vi "WriteReport.vi"(7 "Diag_Ver":string, 8 "error in (no error)":errorcluster, 9 "StepName":string, 10 "Pass/Fail":bool, 11 "GuiRef":T2={"StringOut"=refnum, "AbortOnFail"=refnum, "SN"=refnum, "SN_Length"=refnum, "TestResult"=refnum, "CycleTime"=refnum, "ErrorCode"=refnum, "UUTStatus"=refnum, "DataBaseEnable?"=refnum, "DUTModel"=refnum, "FixtureID"=refnum, "OperatorID"=refnum, "SNReady"=refnum, "StopSlot"=refnum, "NextStep"=refnum, "PassYeild"=refnum, "Failed"=refnum, "Passed"=refnum, "Tested"=refnum, "TestItemsCtl"={"StepName"="", "TestEnable"=FALSE, "LoopCount"=0, "StopOnFail"=FALSE, "Index"=0, "TestName"="", "通道"="", "参数"="", "TimeStart"=0}, "ProcessBar"=refnum, "Slot"=enum."Slot1", "Row"=3, "States"=refnum, "TestMode"=refnum, "循环次数-DUT"=refnum, "波形图"=refnum, "产品型号"=refnum, "子面板"=refnum, "测试失败项目"=refnum, "测试结果"=refnum, "DUT"=refnum, "Starttime"=refnum, "SlotReady"=refnum, "版本信息"=refnum, "WIFI_1"=refnum, "WIFI_2"=refnum, "直通率"=refnum, "卡1开卡结果"=refnum, "卡2开卡结果"=refnum}) -> (0 "error out":errorcluster caption="error out (no error)", 1 "DBresult":bool, 3 "TestData-NHLD":string[](array[string]))   [LabVIEW 2013]
uses:
  SysControl/Reference.ctl
  SysControl/TestItemsCTL.ctl
  SysControl/Slot.ctl
  SourceCode/PDINFO.ctl
  DataBase/DBPara.ctl
  SourceCode/GlobalValue.vi
  <vilib>/Utility/file.llb/Write To Spreadsheet File (string).vi
panel:
  out "Slot":T1
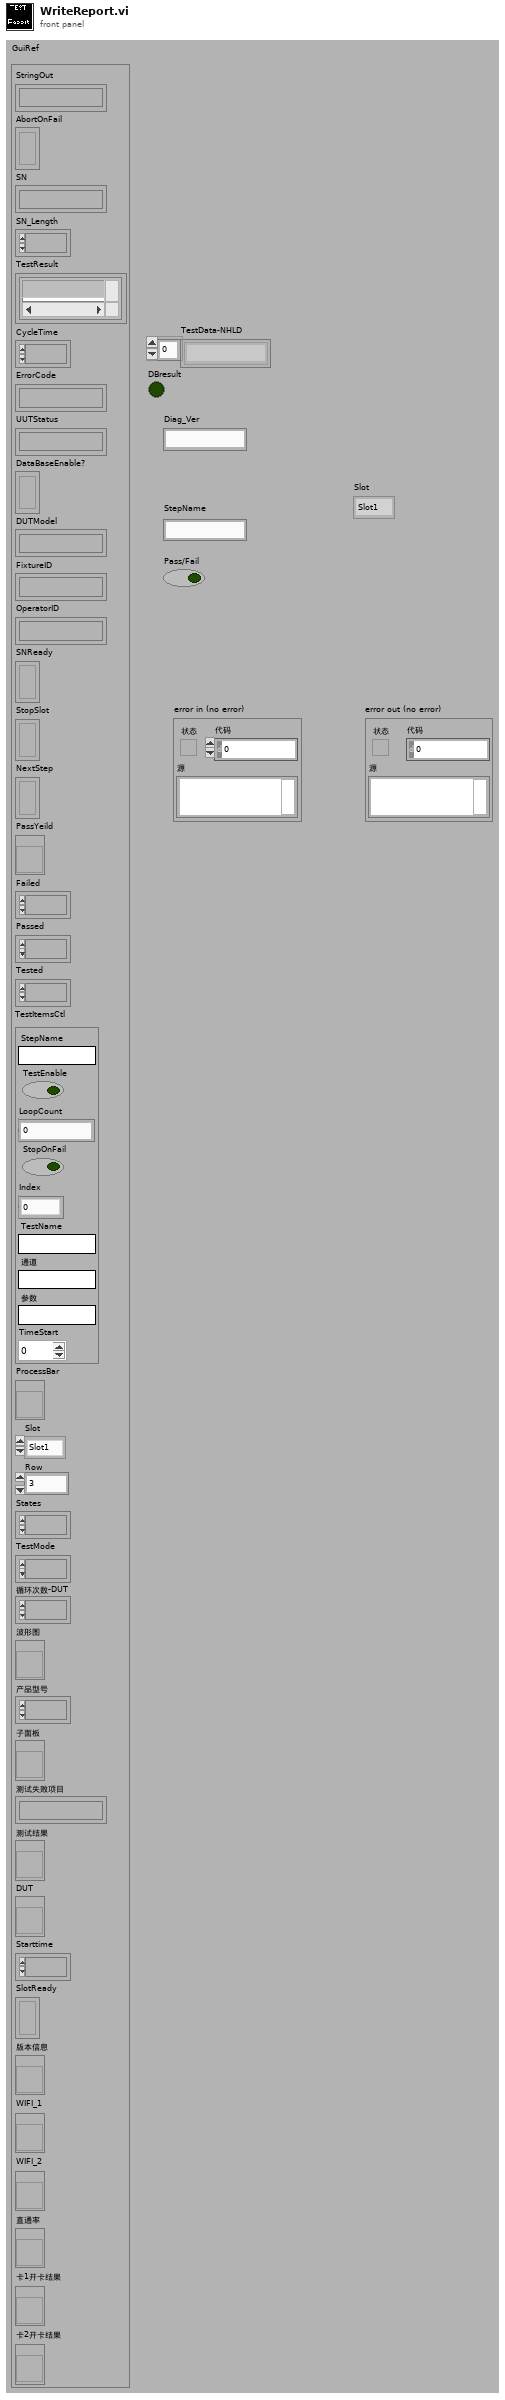
[diagram p1: front panel]
types:
  T1 = typedef "Slot.ctl" = enum16{"Slot1", "Slot2", "Slot3", "Slot4"}
  T2 = typedef "Reference.ctl" = cluster{"StringOut":refnum<vi>, "AbortOnFail":refnum<vi>, "SN":refnum<vi>, "SN_Length":refnum<vi>, "TestResult":refnum<vi>, "CycleTime":refnum<vi>, "ErrorCode":refnum<vi>, "UUTStatus":refnum<vi>, "DataBaseEnable?":refnum<vi>, "DUTModel":refnum<vi>, "FixtureID":refnum<vi>, "OperatorID":refnum<vi>, "SNReady":refnum<vi>, "StopSlot":refnum<vi>, "NextStep":refnum<vi>, "PassYeild":refnum<vi>, "Failed":refnum<vi>, "Passed":refnum<vi>, "Tested":refnum<vi>, "TestItemsCtl":T3, "ProcessBar":refnum<vi>, "Slot":T1, "Row":u32, "States":refnum<vi>, "TestMode":refnum<vi>, "循环次数-DUT":refnum<vi>, "波形图":refnum<vi>, "产品型号":refnum<vi>, "子面板":refnum<vi>, "测试失败项目":refnum<vi>, "测试结果":refnum<vi>, "DUT":refnum<vi>, "Starttime":refnum<vi>, "SlotReady":refnum<vi>, "版本信息":refnum<vi>, "WIFI_1":refnum<vi>, "WIFI_2":refnum<vi>, "直通率":refnum<vi>, "卡1开卡结果":refnum<vi>, "卡2开卡结果":refnum<vi>}
  T3 = typedef "TestItemsCTL.ctl" = cluster{"StepName":string, "TestEnable":bool, "LoopCount":i32, "StopOnFail":bool, "Index":u32, "TestName":string, "通道":string, "参数":string, "TimeStart":u32}
  T4 = enum16{"open", "replace", "create", "open or create", "replace or create", "replace or create with confirmation"}
  T5 = enum16{"Production Mode", "Selection Mode", "Debug Mode", "Loop Mode", "Stop Test"}
  T6 = typedef "PDINFO.ctl" = enum16{"Fw Ver", "HW Ver", "CCID", "WiFiName", "DevID", "SN", "TUID", "CertifID", "PdTime", "Provider", "WiFiPassword", "Imei", "AuthCode", "Reserved1", "Reserved2", "Reserved3"}
  T7 = typedef "DBPara.ctl" = cluster{"DeviceType":string, "PartNumber":string, "TUID":string, "Hw":string, "Sw":string, "PTime":string, "SN":string, "Certid":string, "ICCID":string, "Imei":string, "AuthCode":string, "MAC":string, "Result":string}
  T8 = cluster{"Serial#":string, "TestDate_Time":string, "Operator":string, "TestStation":string, "Fixture#":string, "TestTime":string, "Diag_Ver":string, "Pass_Fail":string}
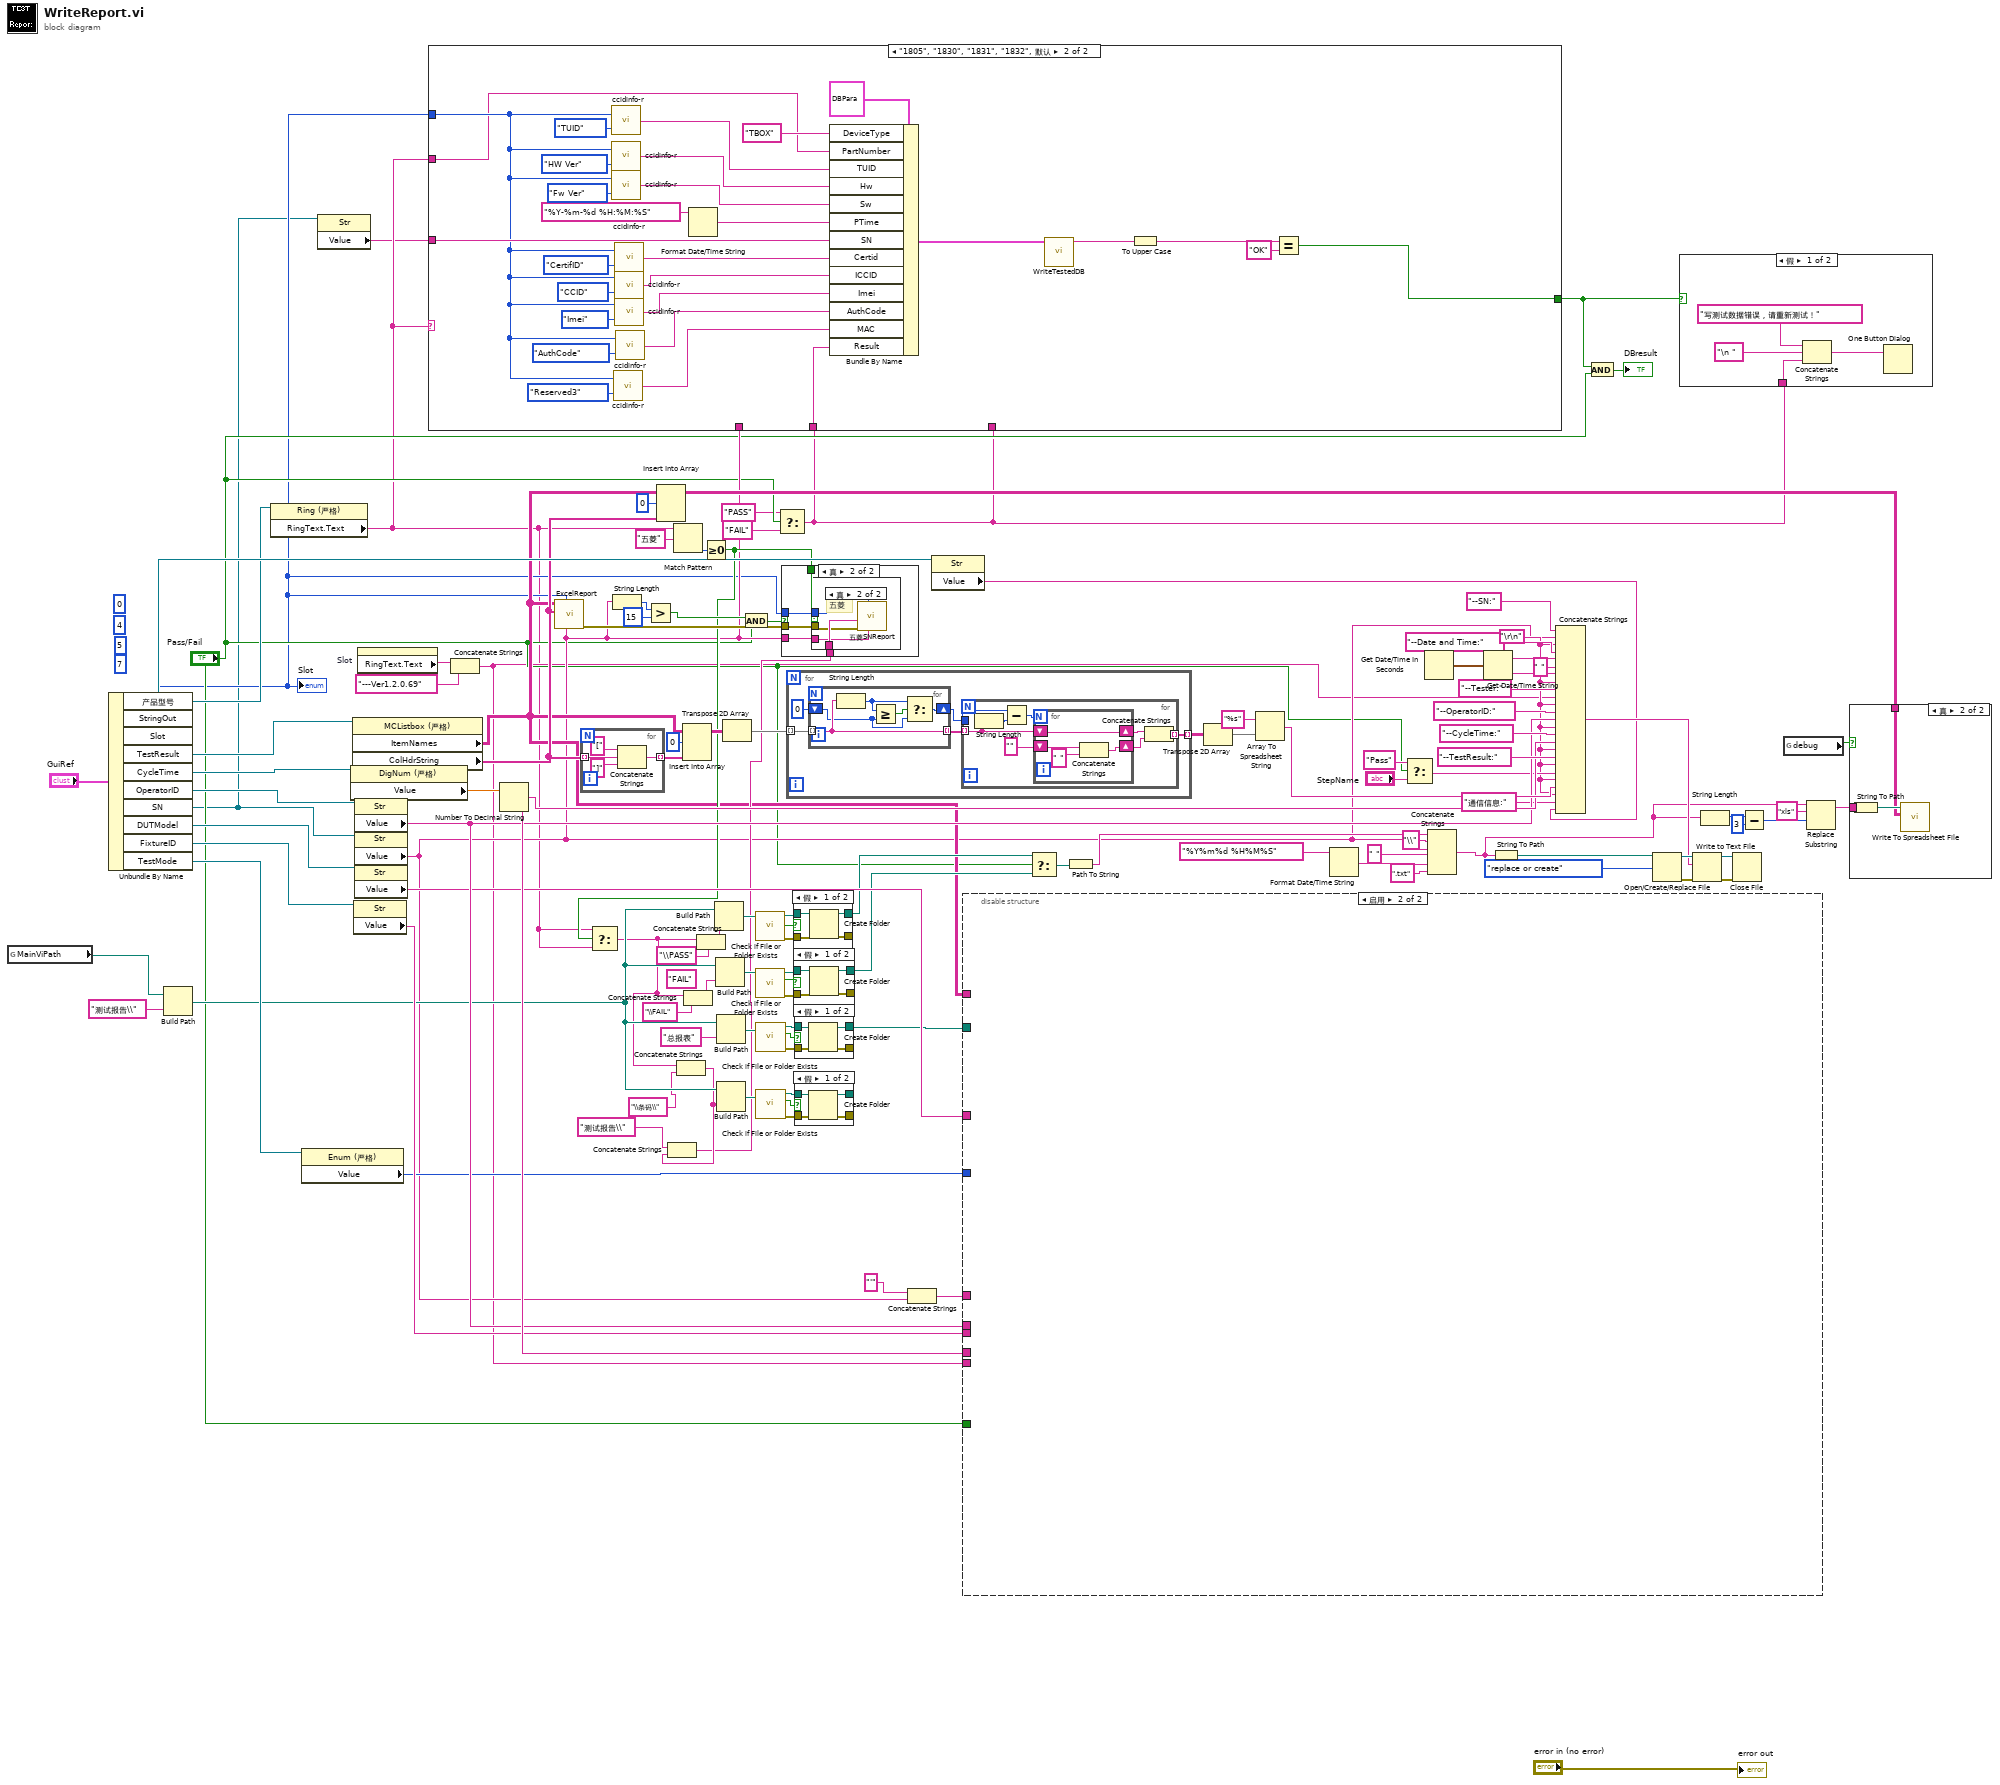
[diagram p0: block diagram]
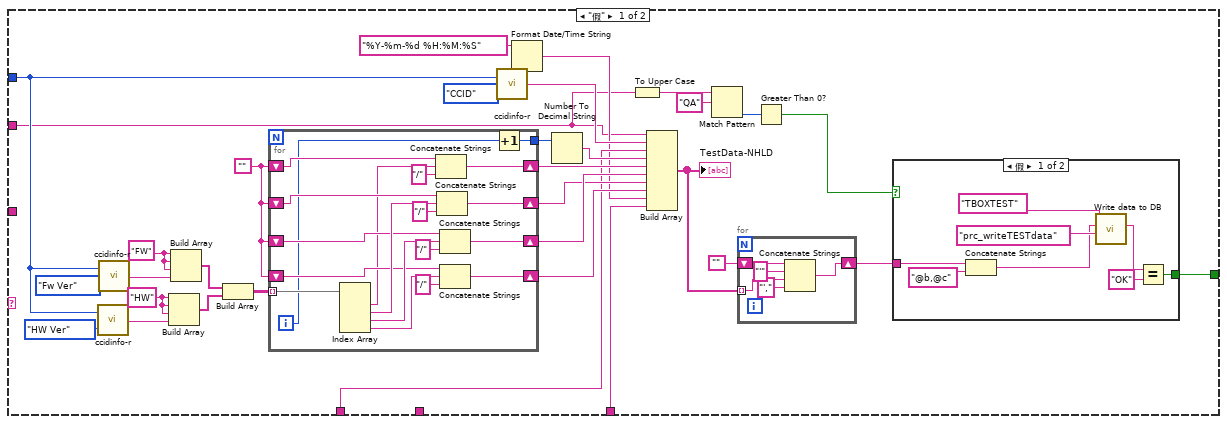
[diagram p2: hidden frame]
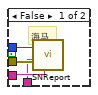
[diagram p7: hidden frame]
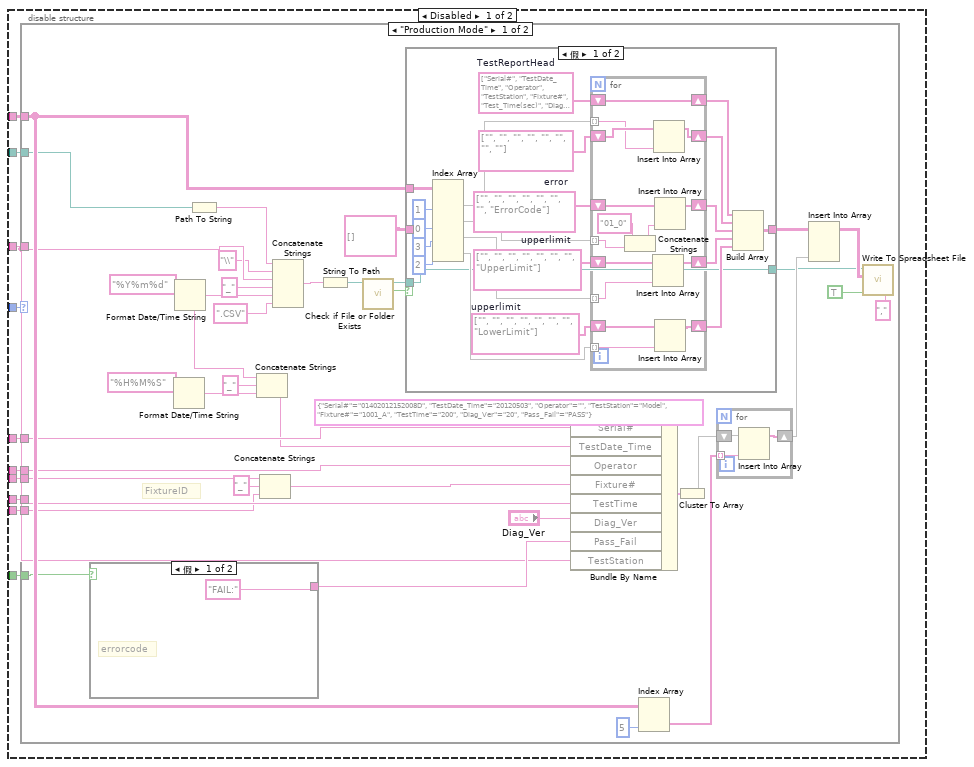
[diagram p9: hidden frame]
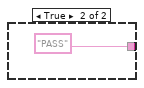
[diagram p10: hidden frame]
diagram:
  (unwired) 7 ("索引")
  (unwired) 5 ("索引")
  (unwired) 4 ("索引")
  (unwired) 0 ("索引")
  (unwired) "FAIL" ("name or relative path")
  w55 = "\r\n"
  n1 = global read "GlobalValue.vi" "MainViPath"() -> (w49:path)
  n2 = Unbundle By Name("GuiRef") -> ("产品型号"=w38:refnum<vi>, "StringOut"=w51:refnum<vi>, "Slot"=w9:T1, "TestResult"=w88:refnum<vi>, "CycleTime"=w87:refnum<vi>, "OperatorID"=w86:refnum<vi>, "SN"=w3:refnum<vi>, "DUTModel"=w85:refnum<vi>, "FixtureID"=w80:refnum<vi>, "TestMode"=w58:refnum<vi>)
  "Slot" <- w9
  n3 = Build Path(base path=w49, name or relative path="测试报告\\" ("名称或相对路径")) -> (appended path=w44:path)
  n4 = property class="Ring (严格)"(reference=w38) -> ("RingText.Text"=w4:string)  [unwired: 1 in, 2 out]
  n5 = property class="Enum (严格)"(reference=w58) -> ("Value"=w57:T5)  [unwired: 1 in, 2 out]
  n6 = property class="Str"(reference=w3) -> ("Value"=w2:string)  [unwired: 1 in, 2 out]
  n7 = property class="DigNum (严格)"(reference=w87) -> ("Value"=w84:dbl)  [unwired: 1 in, 2 out]
  n8 = property class="MCListbox (严格)"(reference=w88) -> ("ItemNames"=w15:string[][], "ColHdrString"=w19:string[])  [unwired: 1 in, 2 out]
  n9 = property class="Str"(reference=w80) -> ("Value"=w79:string)  [unwired: 1 in, 2 out]
  n10 = property class="Str"(reference=w86) -> ("Value"=w83:string)  [unwired: 1 in, 2 out]
  n11 = property class="Str"(reference=w3) -> ("Value"=w14:string)  [unwired: 1 in, 2 out]
  n12 = property class="Str"(reference=w85) -> ("Value"=w82:string)  [unwired: 1 in, 2 out]
  n13 = property on="Slot" class="Enum (严格)"() -> ("RingText.Text"=w7:string)  [unwired: 2 in, 2 out]
  n14 = Concatenate Strings(w7, "---Ver1.2.0.69" ("字符串")) -> (w5:string)
  n15 = Number To Decimal String(number=w84) -> (decimal integer string=w92:string)  [unwired: 1 out]
  n16 = call "ExcelReport.vi"("SN"=w14, "Slot"=w9, "列首字符串"=w19, "TestResults"=w15) -> ("error out"=w43:errorcluster)  [unwired: 7 in]
  n17 = for "For循环" {
    tunnel: w19 -> [w124] mode=indexing
    tunnel: [w122] -> w109 mode=indexing
    n18 = Concatenate Strings("[" ("字符串"), w124, "]" ("字符串")) -> (w122:string)
  }
  n19 = String Length(string=w14) -> (length=w42:i32)
  n20 = Greater?(x=w42, y=15) -> (0:w40:bool)
  n21 = Insert Into Array(array=w15, index (row)=0 ("索引 (行)"), new element=w19) -> (w17:string[][])  [unwired: 1 in]
  n22 = Match Pattern(string=w4, regular expression="五菱" ("正则表达式")) -> (offset past match=w36:i32)  [unwired: 1 in, 3 out]
  n23 = Insert Into Array(array=w15, index (row)=0 ("索引 (行)"), new element=w109) -> (w112:string[][])  [unwired: 1 in]
  n24 = Greater Or Equal To 0?(x=w36) -> (x >= 0?=w35:bool)
  n25 = Select(t=w4, s=w35, f=w4) -> (s? t:f=w29:string)
  n26 = Concatenate Strings(w29, "\\条码\\" ("name or relative path")) -> (w27:string)
  n27 = Concatenate Strings("测试报告\\" ("字符串"), w27) -> (w26:string)
  n28 = Concatenate Strings(w29, "\\FAIL" ("name or relative path")) -> (w31:string)
  n29 = Concatenate Strings(w29, "\\PASS" ("name or relative path")) -> (w34:string)
  n30 = Build Path(base path=w44, name or relative path=w34) -> (appended path=w70:path)
  n31 = Build Path(base path=w44, name or relative path=w31) -> (appended path=w69:path)
  n32 = Build Path(base path=w44, name or relative path="总报表") -> (appended path=w77:path)
  n33 = Build Path(base path=w44, name or relative path=w27) -> (appended path=w46:path)
  n34 = Transpose 2D Array(2D array=w112) -> (transposed array=w120:string[][])
  n35 = And(x=w40, y="Pass/Fail") -> (x .and. y?=w39:bool)
  n36 = call <vilib>:"Check if File or Folder Exists.vi"("path"=w70) -> ("error out"=w74:errorcluster, "file or folder exists?"=w60:bool, "dup path"=w73:path)  [unwired: 1 in, 7 out]
  n37 = call <vilib>:"Check if File or Folder Exists.vi"("path"=w69) -> ("error out"=w71:errorcluster, "file or folder exists?"=w59:bool, "dup path"=w72:path)  [unwired: 1 in, 7 out]
  n38 = call <vilib>:"Check if File or Folder Exists.vi"("path"=w77) -> ("error out"=w76:errorcluster, "file or folder exists?"=w61:bool, "dup path"=w78:path)  [unwired: 1 in, 7 out]
  n39 = call <vilib>:"Check if File or Folder Exists.vi"("path"=w46) -> ("error out"=w47:errorcluster, "file or folder exists?"=w48:bool, "dup path"=w45:path)  [unwired: 1 in, 7 out]
  n40 = Select(t="PASS" ("元素"), s="Pass/Fail", f="FAIL" ("元素")) -> (s? t:f=w1:string)
  n41 = case shown="\"1805\", \"1830\", \"1831\", \"1832\", 默认" w4 {
    tunnel: w14 -> [w150 _]
    tunnel: w9 -> [w139 w200]
    tunnel: w4 -> [w132 w191]
    tunnel: [w129 w192] -> w8
    tunnel: w1 -> [w128 _]
    tunnel: w2 -> [_ w209]
    tunnel: w1 -> [_ w197]
    frame "假" {
      w133 = "HW"
      w134 = "FW"
      w157 = ""
      n42 = call "ccidinfo-r.vi"("Data Type"=PDINFO."HW Ver", "Slot"=w139) -> ("Data"=w138:string)
      n43 = call "ccidinfo-r.vi"("Data Type"=PDINFO."Fw Ver", "Slot"=w139) -> ("Data"=w140:string)
      n44 = Build Array(w133, w133, w133, w138) -> (w136:string[])
      n45 = Build Array(w134, w134, w134, w140) -> (w137:string[])
      n46 = Build Array(w137, w136) -> (w135:string[][])
      n47 = for {
        tunnel: w135 -> [w190] mode=indexing
        shift-right: [w189] -> w156
        shift-left: w157 -> [w188]
        shift-right: [w182] -> w153
        shift-left: w157 -> [w185]
        shift-right: [w180] -> w154
        shift-left: w157 -> [w181]
        shift-right: [w175] -> w155
        shift-left: w157 -> [w177]
        tunnel: [w174] -> w152
        i -> [w173]
        n48 = Index Array(array=w190) -> (element #1=w172:string, element #2=w184:string, element #3=w178:string, element #4=w176:string)  [unwired: 4 in]
        n49 = Concatenate Strings(w188, w172, "/" ("字符串")) -> (w189:string)
        n50 = Concatenate Strings(w185, w184, "/" ("字符串")) -> (w182:string)
        n51 = Concatenate Strings(w181, w178, "/" ("字符串")) -> (w180:string)
        n52 = Concatenate Strings(w177, w176, "/" ("字符串")) -> (w175:string)
        n53 = Increment(x=w173) -> (x+1=w174:i32)
      }
      n54 = call "ccidinfo-r.vi"("Data Type"=PDINFO."CCID", "Slot"=w139) -> ("Data"=w148:string)
      n55 = Format Date/Time String(time format string (%c)="%Y-%m-%d %H:%M:%S" ("时间格式字符串(%c)")) -> (date/time string=w146:string)  [unwired: 2 in]
      n56 = Number To Decimal String(number=w152) -> (decimal integer string=w151:string)  [unwired: 1 in]
      n57 = To Upper Case(1:w132) -> (0:w131:string)
      n58 = Build Array(w132, w148, w150, w151, w156, w154, w153, w155, w146, w128) -> (w145:string[])
      "TestData-NHLD" <- w145
      n59 = Match Pattern(string=w131, regular expression="QA" ("正则表达式")) -> (offset past match=w127:i32)  [unwired: 1 in, 3 out]
      n60 = for {
        tunnel: w145 -> [w169] mode=indexing
        shift-right: [w167] -> w144
        shift-left: "" -> [w171]
        n61 = Concatenate Strings(w171, "'" ("字符串"), w169, "'," ("字符串")) -> (w167:string)
      }
      n62 = Greater Than 0?(x=w127) -> (x > 0?=w126:bool)
      n63 = case shown="假" w126 {
        selector: w126 -> [_ w166]
        tunnel: w144 -> [w165 _]
        tunnel: [w164 w166] -> w129
        frame False {
          n64 = Concatenate Strings(w165, "@b,@c" ("元素")) -> (w159:string)
          n65 = call "Write data to DB.vi"("Procedure name"="prc_writeTESTdata", "all string"=w159, "DSN name"="TBOXTEST") -> ("ResultA"=w161:string)  [unwired: 6 in, 2 out]
          n66 = Equal?(x=w161, y="OK") -> (x = y?=w164:bool)
        }
        frame True {
        }
      }
    }
    frame "1805", "1830", "1831", "1832", Default {
      n67 = call "ccidinfo-r.vi"("Data Type"=PDINFO."TUID", "Slot"=w200) -> ("Data"=w215:string)
      n68 = call "ccidinfo-r.vi"("Data Type"=PDINFO."HW Ver", "Slot"=w200) -> ("Data"=w213:string)
      n69 = call "ccidinfo-r.vi"("Data Type"=PDINFO."Fw Ver", "Slot"=w200) -> ("Data"=w211:string)
      n70 = call "ccidinfo-r.vi"("Data Type"=PDINFO."Reserved3", "Slot"=w200) -> ("Data"=w198:string)
      n71 = call "ccidinfo-r.vi"("Data Type"=PDINFO."CertifID", "Slot"=w200) -> ("Data"=w207:string)
      n72 = call "ccidinfo-r.vi"("Data Type"=PDINFO."CCID", "Slot"=w200) -> ("Data"=w205:string)
      n73 = call "ccidinfo-r.vi"("Data Type"=PDINFO."Imei", "Slot"=w200) -> ("Data"=w203:string)
      n74 = call "ccidinfo-r.vi"("Data Type"=PDINFO."AuthCode", "Slot"=w200) -> ("Data"=w201:string)
      n75 = Format Date/Time String(time format string (%c)="%Y-%m-%d %H:%M:%S" ("时间格式字符串(%c)")) -> (date/time string=w210:string)  [unwired: 2 in]
      n76 = Bundle By Name(cluster=T7 {"DeviceType"="TBOX", "PartNumber"="1805", "TUID"="", "Hw"="Hw", "Sw"="Sw", "PTime"="Sw", "SN"="", "Certid"="", "ICCID"="", "Imei"="", "AuthCode"="", "MAC"="", "Result"=""} ("ParaIn"), "DeviceType"="TBOX", "PartNumber"=w191, "TUID"=w215, "Hw"=w213, "Sw"=w211, "PTime"=w210, "SN"=w209, "Certid"=w207, "ICCID"=w205, "Imei"=w203, "AuthCode"=w201, "MAC"=w198, "Result"=w197) -> (w218:T7)
      n77 = call "WriteTestedDB.vi"("ParaIn"=w218) -> ("ReportStrA"=w194:string)  [unwired: 9 in, 1 out]
      n78 = To Upper Case(1:w194) -> (0:w193:string)
      n79 = Equal?(x=w193, y="OK") -> (x = y?=w192:bool)
    }
  }
  n80 = case shown="真" w39 {
    tunnel: w9 -> [_ w224]
    tunnel: w14 -> [_ w223]
    tunnel: w43 -> [_ w222]
    tunnel: w35 -> [_ w221]
    tunnel: w26 -> [_ w220]
    frame False {
    }
    frame True {
      n81 = case shown="真" w221 {
        tunnel: w224 -> [w228 w229]
        tunnel: w223 -> [w227 w231]
        tunnel: w222 -> [w226 w230]
        tunnel: w220 -> [w225 w232]
        frame False {
          # "海马"
          n82 = call "SNReport.vi"("SN"=w227, "Slot"=w228, "error in (no error)"=w226, "字符串"=w225) -> ()  [unwired: 7 in, 1 out]
        }
        frame True {
          # "五菱"
          n83 = call "五菱SNReport.vi"("SN"=w231, "Slot"=w229, "error in (no error)"=w230, "字符串"=w232) -> ()  [unwired: 7 in, 1 out]
        }
      }
    }
  }
  n84 = for "For循环" {
    tunnel: w120 -> [w235] mode=indexing
    tunnel: [w234] -> w119 mode=indexing
    n85 = for "For循环" {
      tunnel: w235 -> [w254] mode=indexing
      shift-right: [w250] -> w233
      shift-left: 0 -> [w252]
      tunnel: [w254] -> w236 mode=indexing
      n86 = String Length(string=w254) -> (length=w253:i32)
      n87 = Greater Or Equal?(x=w253, y=w252) -> (x >= y?=w251:bool)
      n88 = Select(t=w253, s=w251, f=w252) -> (s? t:f=w250:i32)
    }
    n89 = for "For循环" {
      tunnel: w236 -> [w238] mode=indexing
      tunnel: [w243] -> w234 mode=indexing
      tunnel: w233 -> [w241]
      n90 = String Length(string=w238) -> (length=w245:i32)
      n91 = Subtract(x=w241, y=w245) -> (x-y=w244:i32)
      n92 = for "For循环" {
        N: w244 -> [_]
        shift-right: [w247] -> w240
        shift-left: "" -> [w248]
        shift-right: [w246] -> w239
        shift-left: w238 -> [w246]
        n93 = Concatenate Strings(w248, " ") -> (w247:string)
      }
      n94 = Concatenate Strings(w239, w240) -> (w243:string)
    }
  }
  n95 = case shown="假" w60 {
    tunnel: w73 -> [w258 w259]
    tunnel: [w257 _] -> _
    tunnel: w74 -> [w256 _]
    tunnel: [w255 w259] -> w65
    frame False {
      n96 = Create Folder(path (use dialog)=w258, error in=w256) -> (created path=w255:path, error out=w257:errorcluster)  [unwired: 2 out]
    }
    frame True {
    }
  }
  n97 = case shown="假" w59 {
    tunnel: w72 -> [w263 w264]
    tunnel: [w262 _] -> _
    tunnel: w71 -> [w261 _]
    tunnel: [w260 w264] -> w64
    frame False {
      n98 = Create Folder(path (use dialog)=w263, error in=w261) -> (created path=w260:path, error out=w262:errorcluster)  [unwired: 2 out]
    }
    frame True {
    }
  }
  n99 = case shown="假" w61 {
    tunnel: w78 -> [w268 w269]
    tunnel: [w267 _] -> _
    tunnel: w76 -> [w266 _]
    tunnel: [w265 w269] -> w75
    frame False {
      n100 = Create Folder(path (use dialog)=w268, error in=w266) -> (created path=w265:path, error out=w267:errorcluster)  [unwired: 2 out]
    }
    frame True {
    }
  }
  n101 = case shown="假" w48 {
    tunnel: w45 -> [w273 w274]
    tunnel: [w272 _] -> _
    tunnel: w47 -> [w271 _]
    tunnel: [w270 w274] -> _
    frame False {
      n102 = Create Folder(path (use dialog)=w273, error in=w271) -> (created path=w270:path, error out=w272:errorcluster)  [unwired: 2 out]
    }
    frame True {
    }
  }
  n103 = Concatenate Strings("'" ("string"), w14) -> (w90:string)
  n104 = property class="Str"(reference=w51) -> ("Value"=w50:string)  [unwired: 1 in, 2 out]
  n105 = disable-structure shown="启用" {
    disable-tunnel: w92 -> [w284 _]
    disable-tunnel: w90 -> [w283 _]
    disable-tunnel: w5 -> [w282 _]
    disable-tunnel: w15 -> [w281 _]
    disable-tunnel: w83 -> [w280 _]
    disable-tunnel: w82 -> [w279 _]
    disable-tunnel: w79 -> [w278 _]
    disable-tunnel: w75 -> [w277 _]
    disable-tunnel: w57 -> [w276 _]
    disable-tunnel: "Pass/Fail" -> [w275 _]
    frame Disabled {
      n106 = case shown="\"Production Mode\"" w276 {
        tunnel: w281 -> [w318 _]
        tunnel: w283 -> [w306 _]
        tunnel: w275 -> [w309 _]
        tunnel: w282 -> [w288 _]
        tunnel: w284 -> [w294 _]
        tunnel: w280 -> [w297 _]
        tunnel: w279 -> [w291 _]
        tunnel: w278 -> [w286 _]
        tunnel: w277 -> [w285 _]
        frame "Production Mode" {
          # "FixtureID"
          n107 = case shown="假" w309 {
            tunnel: ["FAIL:" ("TesterID") "PASS" ("TesterID")] -> w292
            frame False {
              # "errorcode"
            }
            frame True {
            }
          }
          n108 = Format Date/Time String(time format string (%c)="%H%M%S") -> (date/time string=w299:string)  [unwired: 2 out]
          n109 = Format Date/Time String(time format string (%c)="%Y%m%d") -> (date/time string=w300:string)  [unwired: 2 out]
          n110 = Path To String(path=w285) -> (string=w289:string)
          n111 = Concatenate Strings(w300, "_" ("string"), w299) -> (w298:string)
          n112 = Concatenate Strings(w286, "_" ("string"), w288) -> (w295:string)
          n113 = Concatenate Strings(w289, "\\" ("字符串"), w291, "_", w300, ".CSV" ("字符串")) -> (w311:string)
          n114 = String To Path(string=w311) -> (path=w304:path)
          n115 = call <vilib>:"Check if File or Folder Exists.vi"("path"=w304) -> ("file or folder exists?"=w315:bool, "dup path"=w303:path)  [unwired: 1 in, 8 out]
          n116 = case shown="假" w315 {
            tunnel: [w344 w363] -> w321
            tunnel: w318 -> [w329 _]
            tunnel: string[][] [] ("数组 2") -> [_ w363]
            tunnel: w303 -> [w326 w362]
            tunnel: [w326 w362] -> w287
            frame False {
              w339 = string[] ["", "", "", "", "", "", "", "LowerLimit"]  # upperlimit
              w341 = string[] ["", "", "", "", "", "", "", "UpperLimit"]  # upperlimit
              w342 = string[] ["", "", "", "", "", "", "", "ErrorCode"]  # error
              w346 = string[] ["Serial#", "TestDate_Time", "Operator", "TestStation", "Fixture#", "Test_Time(sec)", "Diag_Ver", "Pass_Fail", "NAME", ""]  # TestReportHead
              n117 = Index Array(array=w329, index (col) #1=1 ("禁用的索引 (列)"), index (col) #2=0 ("索引 (列)"), index (col) #3=3 ("索引 (列)"), index (col) #4=2 ("索引 (列)")) -> (element #1=w332:string[], element #2=w333:string[], element #3=w328:string[], element #4=w327:string[])  [unwired: 4 in]
              n118 = for {
                shift-right: [w350] -> w345
                shift-left: w346 -> [w350]
                tunnel: w332 -> [w351] mode=indexing
                shift-right: [w360] -> w343
                shift-left: w342 -> [w361]
                tunnel: w333 -> [w348] mode=indexing
                tunnel: w328 -> [w359] mode=indexing
                shift-right: [w357] -> w340
                shift-left: w341 -> [w358]
                shift-right: [w356] -> w338
                shift-left: w339 -> [w355]
                tunnel: w327 -> [w354] mode=indexing
                shift-right: [w352] -> w336
                shift-left: string[] ["", "", "", "", "", "", "", ""] -> [w353]
                n119 = Concatenate Strings("01_0" ("string"), w348) -> (w347:string)
                n120 = Insert Into Array(array=w358, new element=w359) -> (w357:string[])  [unwired: 1 in]
                n121 = Insert Into Array(array=w353, new element=w351) -> (w352:string[])  [unwired: 1 in]
                n122 = Insert Into Array(array=w361, new element=w347) -> (w360:string[])  [unwired: 1 in]
                n123 = Insert Into Array(array=w355, new element=w354) -> (w356:string[])  [unwired: 1 in]
              }
              n124 = Build Array(w345, w336, w343, w340, w338) -> (w344:string[][])
            }
            frame True {
            }
          }
          n125 = Bundle By Name(cluster=T8 {"Serial#"="01402012152008D", "TestDate_Time"="20120503", "Operator"="", "TestStation"="Model", "Fixture#"="1001_A", "TestTime"="200", "Diag_Ver"="20", "Pass_Fail"="PASS"} ("output cluster"), "Serial#"=w306, "TestDate_Time"=w298, "Operator"=w297, "Fixture#"=w295, "TestTime"=w294, "Diag_Ver"="Diag_Ver", "Pass_Fail"=w292, "TestStation"=w291) -> (w308:T8)
          n126 = Index Array(array=w318, index (col)=5 ("索引 (列)")) -> (element=w319:string[])  [unwired: 1 in]
          n127 = Cluster To Array(cluster=w308) -> (array=w323:string[])
          n128 = for {
            tunnel: w319 -> [w365] mode=indexing
            shift-right: [w364] -> w322
            shift-left: w323 -> [w366]
            n129 = Insert Into Array(array=w366, new element=w365) -> (w364:string[])  [unwired: 1 in]
          }
          n130 = Insert Into Array(array=w321, new element=w322) -> (w314:string[][])  [unwired: 2 in]
          n131 = call-poly <vilib>:"Write To Spreadsheet File.vi"("delimiter (\\t)"="," ("delimiter (\\t)"), "append to file? (new file:F)"=TRUE, "2D data"=w314, "file path (dialog if empty)"=w287) -> ()  [unwired: 3 in, 2 out]
        }
        frame "Debug Mode", Default {
        }
      }
    }
    frame Enabled {
    }
  }
  n132 = Select(t=w65, s="Pass/Fail", f=w64) -> (s? t:f=w63:path)
  n133 = Path To String(path=w63) -> (string=w62:string)
  n134 = Transpose 2D Array(2D array=w119) -> (transposed array=w113:string[][])
  n135 = Array To Spreadsheet String(array=w113, 3:"%s" ("format string")) -> (spreadsheet string=w116:string)  [unwired: 1 out]
  n136 = Format Date/Time String(time format string (%c)="%Y%m%d %H%M%S") -> (date/time string=w102:string)  [unwired: 2 out]
  n137 = Select(t="Pass", s="Pass/Fail", f="StepName") -> (s? t:f=w66:string)
  n138 = Get Date/Time In Seconds() -> (seconds since 1Jan1904=w115:timestamp)
  n139 = Concatenate Strings(w62, "\\" ("string"), w14, " " ("string"), w102, ".txt" ("字符串")) -> (w23:string)
  n140 = Get Date/Time String(seconds (now)=w115) -> (date string=w98:string, time string=w96:string)  [unwired: 2 out]
  n141 = String To Path(string=w23) -> (path=w108:path)
  n142 = Concatenate Strings("--SN:" ("element"), w14, w55, "--Date and Time:" ("元素"), w98, " " ("字符串"), w96, w55, "--Tester:" ("element"), w5, w55, "--OperatorID:" ("string"), w83, w55, "--CycleTime:" ("字符串"), w92, w55, "--TestResult:" ("元素"), w55, w66, w55, w116, w55, "通信信息:" ("字符串"), w50) -> (w104:string)
  n143 = And(x=w8, y="Pass/Fail") -> (x .and. y?=→"DBresult":bool)
  n144 = Open/Create/Replace File(file path (use dialog)=w108, operation (0:open)=T4."replace or create" ("操作(0:open)")) -> (refnum out=w107:refnum<file>, error out=w105:errorcluster)  [unwired: 1 in, 4 out]
  n145 = case shown="假" w8 {
    tunnel: w1 -> [w368 _]
    frame False {
      n146 = Concatenate Strings("写测试数据错误，请重新测试！" ("消息"), "\n ", w368) -> (w367:string)
      n147 = One Button Dialog(message=w367) -> ()  [unwired: 1 in, 1 out]
    }
    frame True {
    }
  }
  n148 = Write to Text File(file (use dialog)=w107, text=w104, error in=w105) -> (refnum out=w110:refnum<file>, error out=w111:errorcluster)  [unwired: 2 out]
  n149 = String Length(string=w23) -> (length=w25:i32)
  n150 = Close File(refnum=w110, error in=w111) -> ()  [unwired: 2 out]
  n151 = Subtract(x=w25, y=3) -> (x-y=w21:i32)
  n152 = global read "GlobalValue.vi" "debug"() -> (w16:bool)
  n153 = Replace Substring(3:w21, 4:"xls" ("子字符串(\"\")"), 5:w23) -> (1:w20:string)  [unwired: 1 in, 1 out]
  n154 = case shown="真" w16 {
    tunnel: w20 -> [_ w373]
    tunnel: w17 -> [_ w371]
    frame False {
    }
    frame True {
      n155 = String To Path(string=w373) -> (path=w372:path)
      n156 = call-poly <vilib>:"Write To Spreadsheet File.vi"("2D data"=w371, "file path (dialog if empty)"=w372) -> ()  [unwired: 6 in, 1 out]
    }
  }
  "error out" <- "error in (no error)"
